vi "PathPlanner_Cmd_AutoRamseteExecute.vi"(5 "PathPlanner_Cmd_FollowRamConfig":T18={"ControlPastEnd_Sec"=3.0, "Trigger Events"=TRUE, "RAMSETE_EXE_TUNING SI"={"B"=2.0, "Zeta"=0.7, "X Tolerance M"=2.0, "Y Tolerance M"=0.7, "Heading Tolerance RAD"=0.7, "Track Width M"=2.0, "Max Speed M/S"=2.0}} {"RAMSETE_EXE_TUNING SI"."Max Speed M/S" format="%13.4f"; "RAMSETE_EXE_TUNING SI"."Track Width M" format="%13.4f"; "RAMSETE_EXE_TUNING SI"."Heading Tolerance RAD" format="%13.4f"; "RAMSETE_EXE_TUNING SI"."Y Tolerance M" format="%13.4f"; "RAMSETE_EXE_TUNING SI"."X Tolerance M" format="%13.4f"; "RAMSETE_EXE_TUNING SI"."Zeta" format="%13.4f"; "RAMSETE_EXE_TUNING SI"."B" format="%13.4f"}, 6 "PassthroughTime_SEC":dbl=-1.0, 7 "PathPlanner_Cmd_AutoConfig":T3 {"Paths"."IdealStartingState"."Rotation"."SIN" format="%13.4f"; "Paths"."IdealStartingState"."Rotation"."COS" format="%13.4f"; "Paths"."IdealStartingState"."Rotation"."VALUE" format="%13.4f"; "Paths"."PointTowardsZones"."TargetPosition"."Y" format="%14.3f"; "Paths"."PointTowardsZones"."TargetPosition"."X" format="%14.3f"; "Paths"."PointTowardsZones"."RotationOffset"."SIN" format="%13.4f"; "Paths"."PointTowardsZones"."RotationOffset"."COS" format="%13.4f"; "Paths"."PointTowardsZones"."RotationOffset"."VALUE" format="%13.4f"; "Paths"."Waypoints"."nextControl"."Y" format="%14.3f"; "Paths"."Waypoints"."nextControl"."X" format="%14.3f"; "Paths"."Waypoints"."anchor"."Y" format="%14.3f"; "Paths"."Waypoints"."anchor"."X" format="%14.3f"; "Paths"."Waypoints"."prevControl"."Y" format="%14.3f"; "Paths"."Waypoints"."prevControl"."X" format="%14.3f"; "Paths"."AllPoints"."RotationTarget"."rotation"."SIN" format="%13.4f"; "Paths"."AllPoints"."RotationTarget"."rotation"."COS" format="%13.4f"; "Paths"."AllPoints"."RotationTarget"."rotation"."VALUE" format="%13.4f"; "Paths"."AllPoints"."Position"."Y" format="%14.3f"; "Paths"."AllPoints"."Position"."X" format="%14.3f"; "Paths"."GoalEndState"."Rotation"."SIN" format="%13.4f"; "Paths"."GoalEndState"."Rotation"."COS" format="%13.4f"; "Paths"."GoalEndState"."Rotation"."VALUE" format="%13.4f"; "Paths"."RotationTargets"."rotation"."SIN" format="%13.4f"; "Paths"."RotationTargets"."rotation"."COS" format="%13.4f"; "Paths"."RotationTargets"."rotation"."VALUE" format="%13.4f"}, 8 "Enabled":bool=TRUE, 9 "Reset":bool, 10 "CurrentChassisSpeeds":T2 {"vOmega" format="%10.3f"; "vY" format="%10.3f"; "vX" format="%10.3f"}, 11 "Current Pose SI":T20={"TRANSLATION"={"X"=0.0, "Y"=0.0}, "ROTATION"={"VALUE"=0.0, "COS"=1.0, "SIN"=0.0}} {"ROTATION"."SIN" format="%13.4f"; "ROTATION"."COS" format="%13.4f"; "ROTATION"."VALUE" format="%13.4f"; "TRANSLATION"."Y" format="%14.3f"; "TRANSLATION"."X" format="%14.3f"}) -> (0 "Position Error M":dbl, 1 "Complete":bool, 2 "At Reference":bool, 3 "Left Right Speed Dmds":T1)   [LabVIEW 2019, in "PathPlanner24.lvlib"]
doc: "DOCUMENTATION IS NOT COMPLETE.\n \nCalculates the next output of the path following controller for holonomic drive robots. This wraps a Holonomic Drive Control function with the particulars needed to follow a PathPlanner trajectory.\n\nInputs:\n - PathPlanner_Holonomic_Ctrl_Pack_Tuning - cluster - The tuning paraameters for the holonomic drive controller. These are static. They should not be changed after the first call to this function.\n - CurrentPoseSi - pose2d - The current pose calculated by odometry or pose estimation. The pose can be absolute or relative depending on what type of trajectory is being followed.\n - PathPlannerState - cluster - The path palnner trajectory state containing the desired position and velocities of the robot.\n - Reset - boolean - When TRUE the holonomic drive controller is reset. This should be set to TRUE for the first execution of a trajectory.\n - Enabled - boolean - When TRUE, closed loop control is enabled. (Optional. Default: TRUE)\n - Period - double - The loop period in seconds for this controller. (Optional. Default: 0.020)\n\nOutputs:\n - CalcChassisSpeed - cluster - The desired chassis speed in SI units.\n - AtReference - boolean - TRUE if the robots position is within the defined tolerance.\n - PositionError - pose2d - Position error in SI units. How far the robot is away from the desired trajectory position.\n - out_Holonomic_Drive_Ctrl - THe current holonomic drive controller data cluster. This is mainly for diagnostic purposes."
uses:
  PathPlanner24.lvlib
  <vilib>/Rock Robotics/WPI/ThirdParty/JAS_Junk/TrajLib/TypeDef/TRANSLATION2D.ctl
  <vilib>/Rock Robotics/WPI/ThirdParty/JAS_Junk/TrajLib/Trajectory_Library.lvlib
  <vilib>/Rock Robotics/WPI/ThirdParty/JAS_Junk/TrajLib/TypeDef/ROTATION2D.ctl
  <vilib>/Rock Robotics/WPI/ThirdParty/JAS_Junk/TrajLib/TypeDef/POSE2D.ctl
  <vilib>/Rock Robotics/WPI/ThirdParty/JAS_Junk/TrajLib/TypeDef/CHASSIS_SPEEDS.ctl
  TypeDef/PathPlannerRotationTarget.ctl
  TypeDef/PathPlannerPathConstraints.ctl
  TypeDef/PathPlannerConstraintsZone.ctl
  TypeDef/PathPlannerCommandUtil.ctl
  TypeDef/PathPlannerEventMarker.ctl
  TypeDef/PathPlannerGoalEndState.ctl
  TypeDef/PathPlannerPathPoint.ctl
  TypeDef/PathPlannerPath.ctl
  TypeDef/PathPlannerWaypoint.ctl
  TypeDef/PathPlannerPointTowardsZone.ctl
  TypeDef/PathPlannerIdealStartingState.ctl
  TypeDef/PathPlannerCmdPathPlannerAutoConfig.ctl
  <vilib>/Rock Robotics/WPI/ThirdParty/JAS_Junk/TrajLib/TypeDef/RAMSETE_EXE_TUNING.ctl
  TypeDef/PathPlannerCmdFollowRamConfig.ctl
  ENum/PathPlanner_CommandUtil_Type_ENUM.ctl
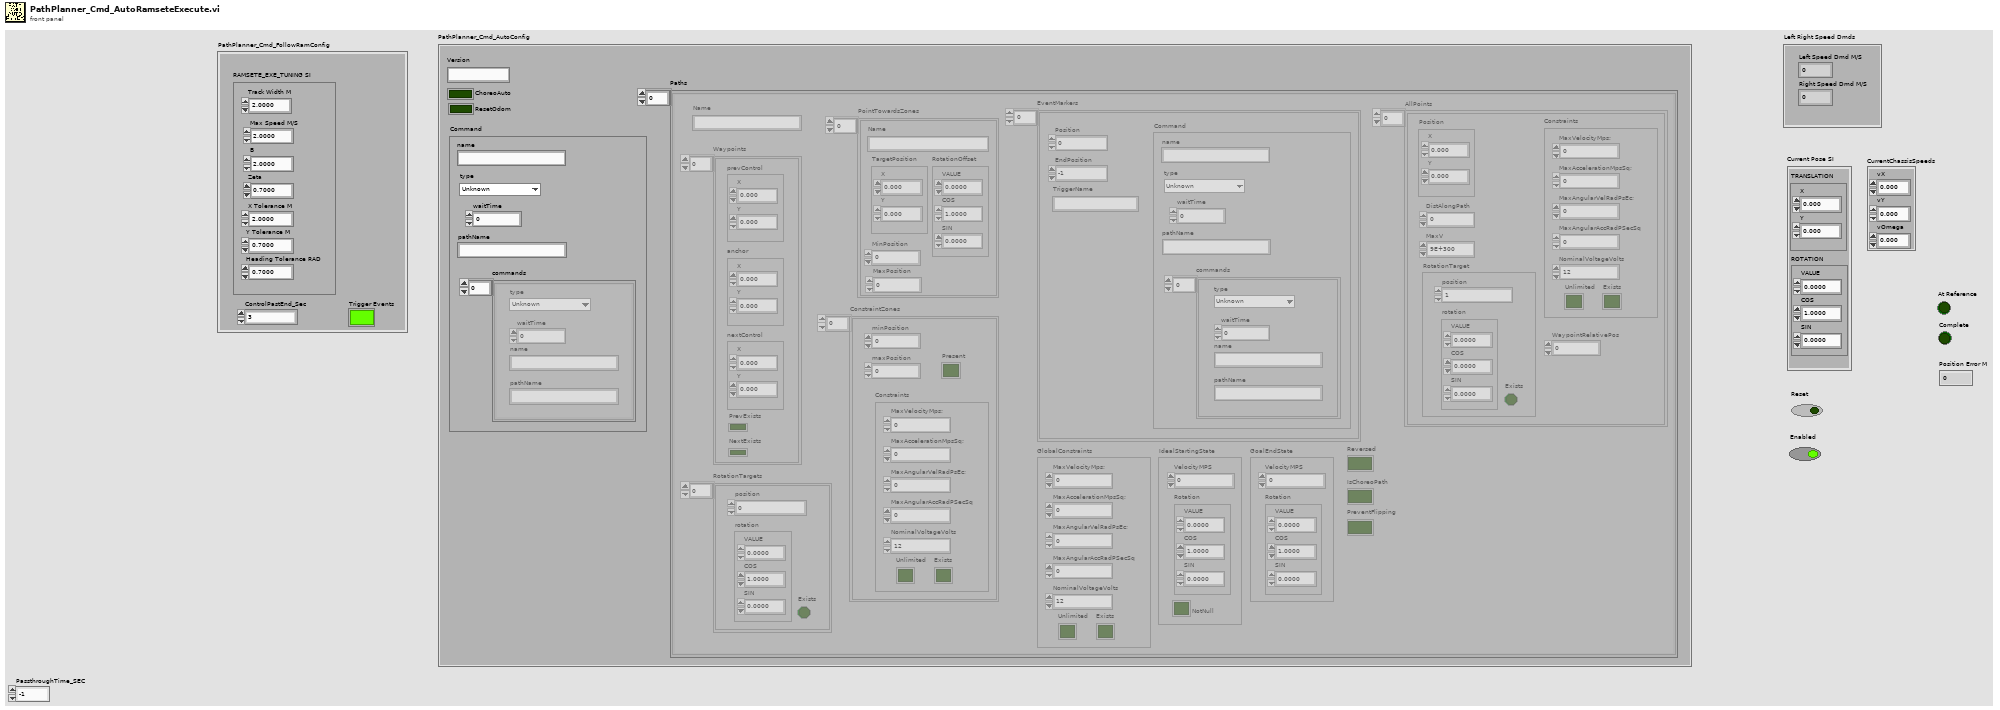
[diagram p1: front panel]
types:
  T1 = cluster{"Left Speed Dmd M/S":dbl, "Right Speed Dmd M/S":dbl}
  T2 = typedef "Trajectory_Library.lvlib/CHASSIS_SPEEDS.ctl" = cluster{"vX":dbl, "vY":dbl, "vOmega":dbl}
  T3 = typedef "PathPlanner24.lvlib/PathPlannerCmdPathPlannerAutoConfig.ctl" = cluster{"Command":T4, "ChoreoAuto":bool, "Version":string, "ResetOdom":bool, "Paths":T6[]}
  T4 = typedef "PathPlanner24.lvlib/PathPlannerCommandUtil.ctl" = cluster{"waitTime":dbl, "name":string, "pathName":string, "commands":cluster{"type":T5, "waitTime":dbl, "name":string, "pathName":string}[], "type":T5}
  T5 = typedef "PathPlanner24.lvlib/PathPlanner_CommandUtil_Type_ENUM.ctl" = enum16{"Unknown", "Wait", "Named", "Path", "Sequential", "Parallel", "Race", "Deadline", "PointTowardsZoneEnter", "PointTowardsZoneExit", "TriggerEventStart", "TriggerEventStop", "TriggerEventOneshot"}
  T6 = typedef "PathPlanner24.lvlib/PathPlannerPath.ctl" = cluster{"Reversed":bool, "RotationTargets":T7[], "ConstraintZones":T9[], "EventMarkers":T11[], "GlobalConstraints":T10, "GoalEndState":T12, "AllPoints":T13[], "Name":string, "Waypoints":T15[], "PointTowardsZones":T16[], "IdealStartingState":T17, "IsChoreoPath":bool, "PreventFlipping":bool}
  T7 = typedef "PathPlanner24.lvlib/PathPlannerRotationTarget.ctl" = cluster{"position":dbl, "rotation":T8, "Exists":bool}
  T8 = typedef "Trajectory_Library.lvlib/ROTATION2D.ctl" = cluster{"VALUE":dbl, "COS":dbl, "SIN":dbl}
  T9 = typedef "PathPlanner24.lvlib/PathPlannerConstraintsZone.ctl" = cluster{"minPosition":dbl, "maxPosition":dbl, "Constraints":T10, "Present":bool}
  T10 = typedef "PathPlanner24.lvlib/PathPlannerPathConstraints.ctl" = cluster{"MaxVelocityMps;":dbl, "MaxAccelerationMpsSq;":dbl, "MaxAngularVelRadPsEc;":dbl, "MaxAngularAccRadPSecSq":dbl, "Exists":bool, "Unlimited":bool, "NominalVoltageVolts":dbl}
  T11 = typedef "PathPlanner24.lvlib/PathPlannerEventMarker.ctl" = cluster{"Position":dbl, "Command":T4, "TriggerName":string, "EndPosition":dbl}
  T12 = typedef "PathPlanner24.lvlib/PathPlannerGoalEndState.ctl" = cluster{"VelocityMPS":dbl, "Rotation":T8}
  T13 = typedef "PathPlanner24.lvlib/PathPlannerPathPoint.ctl" = cluster{"Position":T14, "DistAlongPath":dbl, "MaxV":dbl, "Constraints":T10, "RotationTarget":T7, "WaypointRelativePos":dbl}
  T14 = typedef "Trajectory_Library.lvlib/TRANSLATION2D.ctl" = cluster{"X":dbl, "Y":dbl}
  T15 = typedef "PathPlanner24.lvlib/PathPlannerWaypoint.ctl" = cluster{"prevControl":T14, "anchor":T14, "nextControl":T14, "PrevExists":bool, "NextExists":bool}
  T16 = typedef "PathPlanner24.lvlib/PathPlannerPointTowardsZone.ctl" = cluster{"RotationOffset":T8, "Name":string, "TargetPosition":T14, "MinPosition":dbl, "MaxPosition":dbl}
  T17 = typedef "PathPlanner24.lvlib/PathPlannerIdealStartingState.ctl" = cluster{"VelocityMPS":dbl, "Rotation":T8, "NotNull":bool}
  T18 = typedef "PathPlanner24.lvlib/PathPlannerCmdFollowRamConfig.ctl" = cluster{"ControlPastEnd_Sec":dbl, "Trigger Events":bool, "RAMSETE_EXE_TUNING SI":T19}
  T19 = typedef "Trajectory_Library.lvlib/RAMSETE_EXE_TUNING.ctl" = cluster{"B":dbl, "Zeta":dbl, "X Tolerance M":dbl, "Y Tolerance M":dbl, "Heading Tolerance RAD":dbl, "Track Width M":dbl, "Max Speed M/S":dbl}
  T20 = typedef "Trajectory_Library.lvlib/POSE2D.ctl" = cluster{"TRANSLATION":T14, "ROTATION":T8}
  T21 = cluster{"type":T5, "waitTime":dbl, "name":string, "pathName":string}[]
  T22 = cluster{"type":T5, "waitTime":dbl, "name":string, "pathName":string}
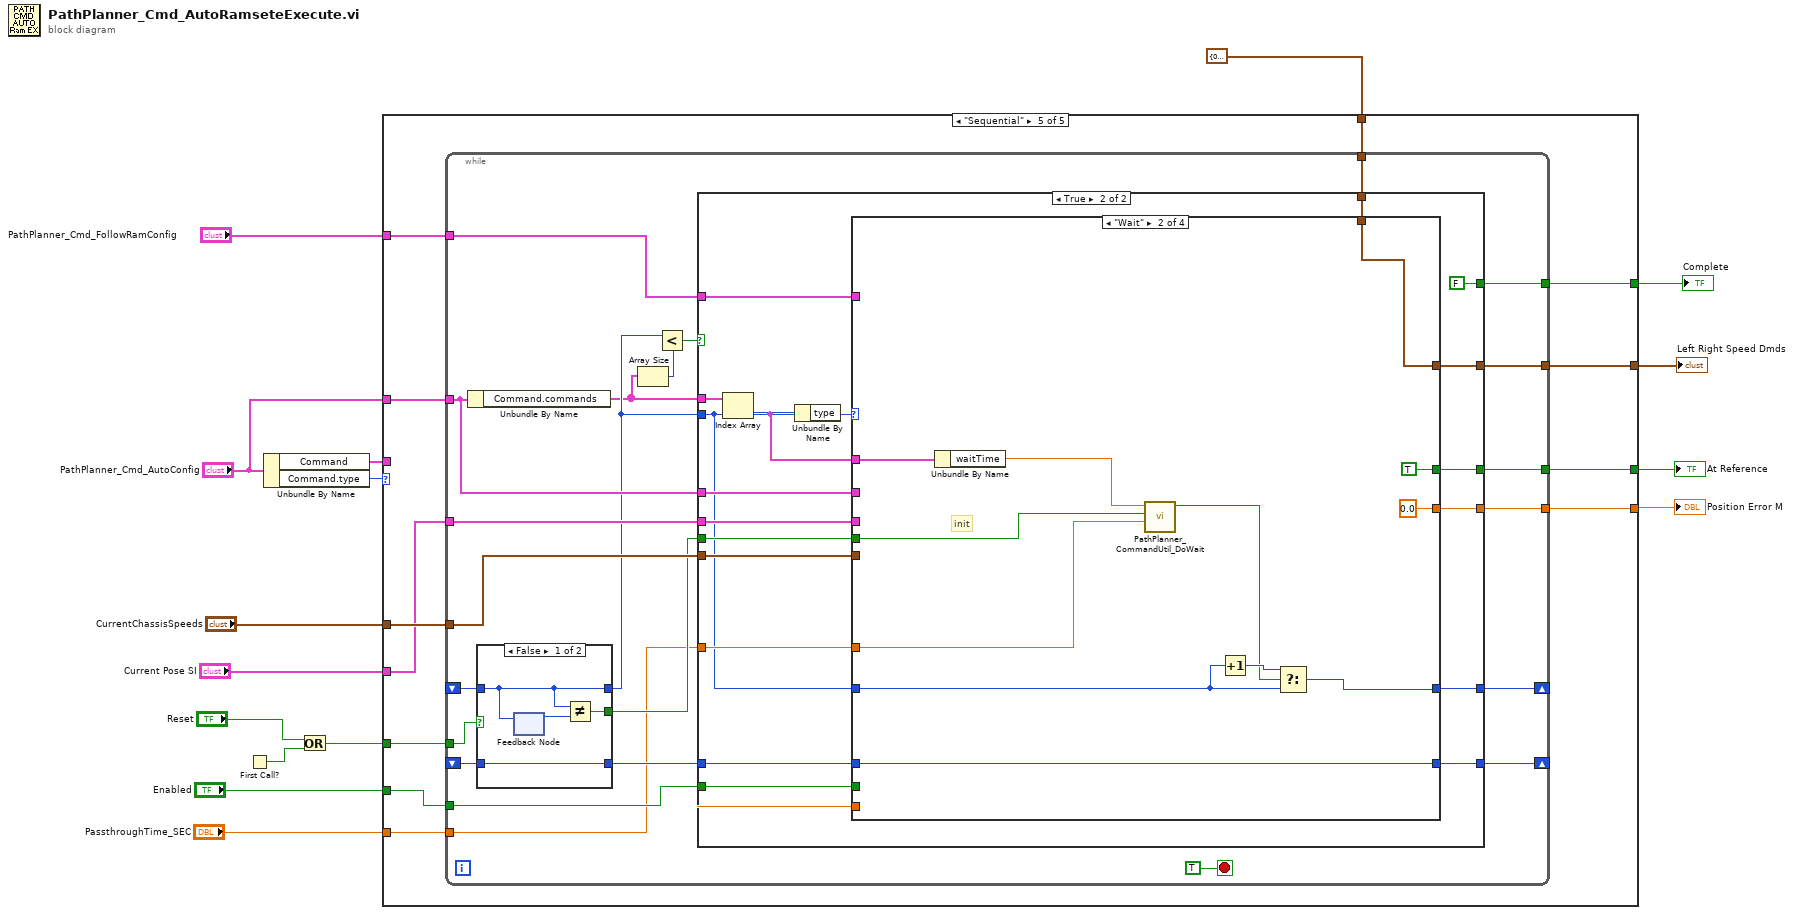
[diagram p0: block diagram]
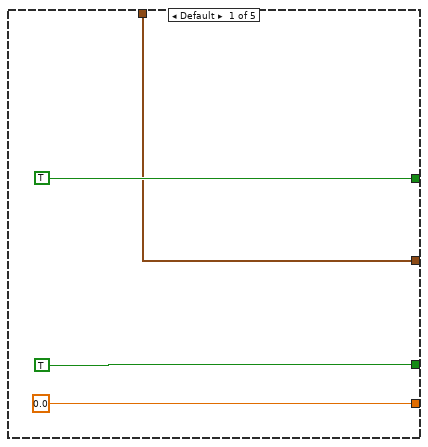
[diagram p2: hidden frame]
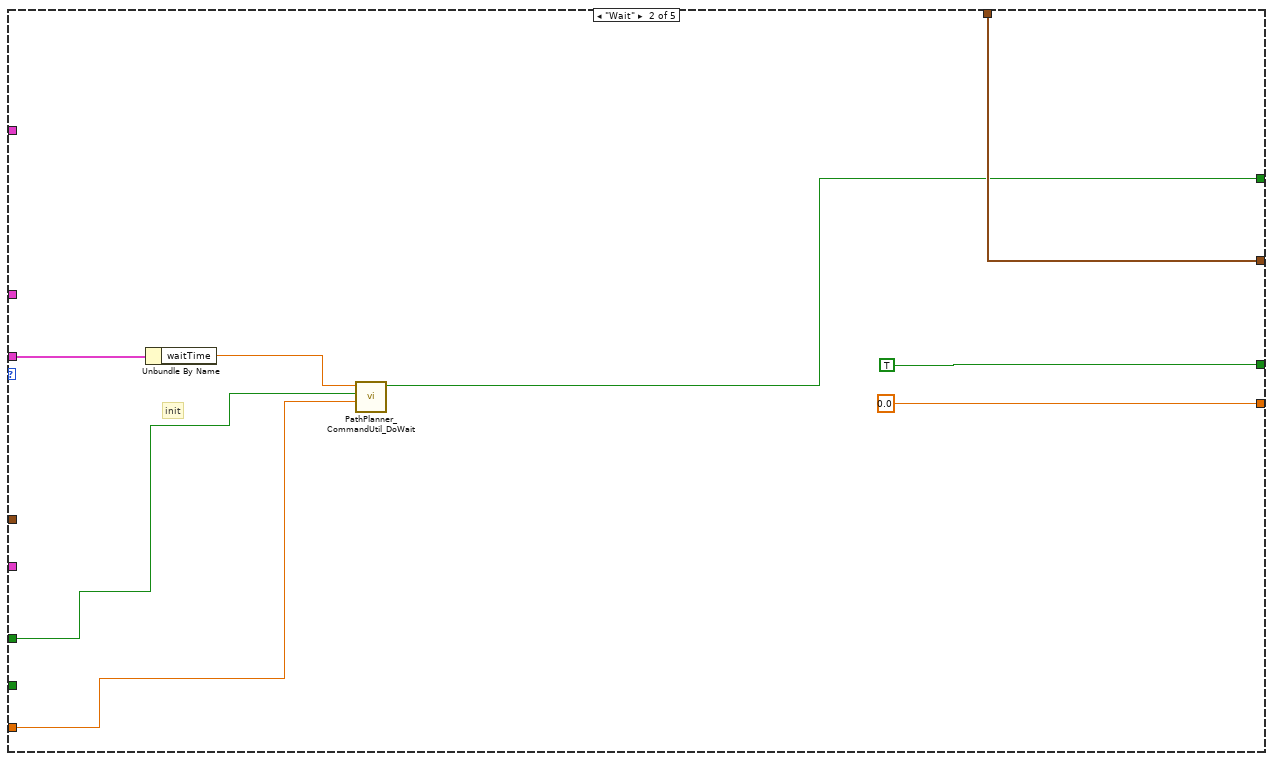
[diagram p3: hidden frame]
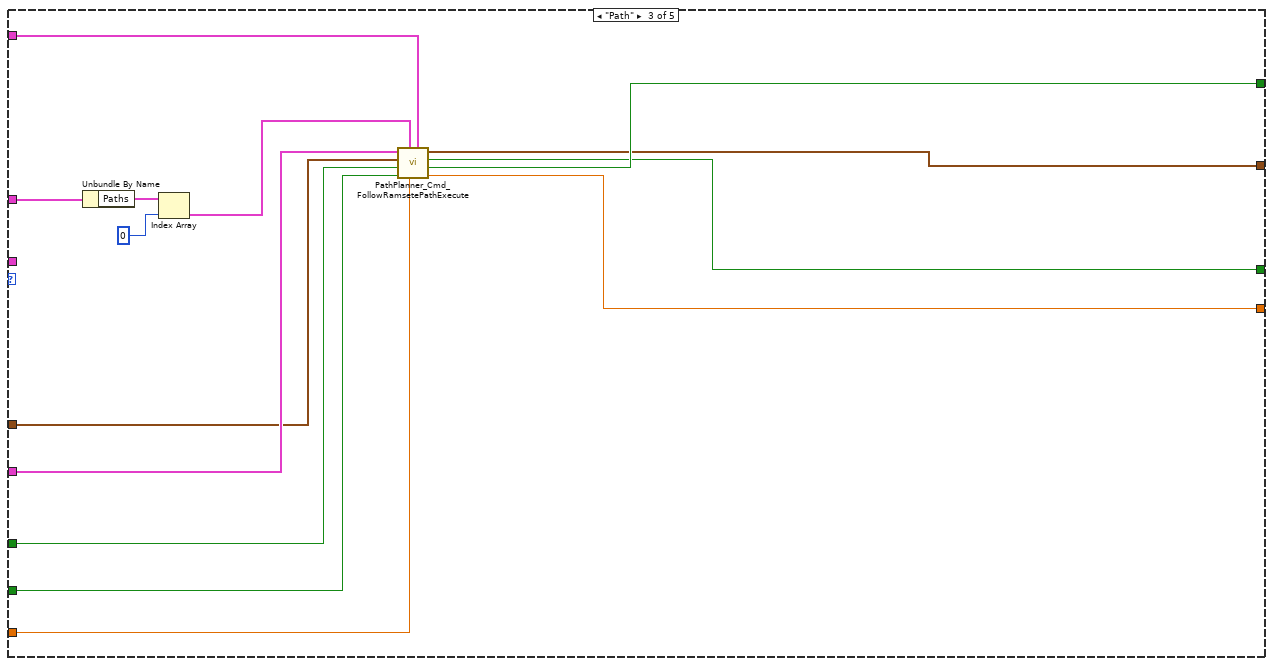
[diagram p4: hidden frame]
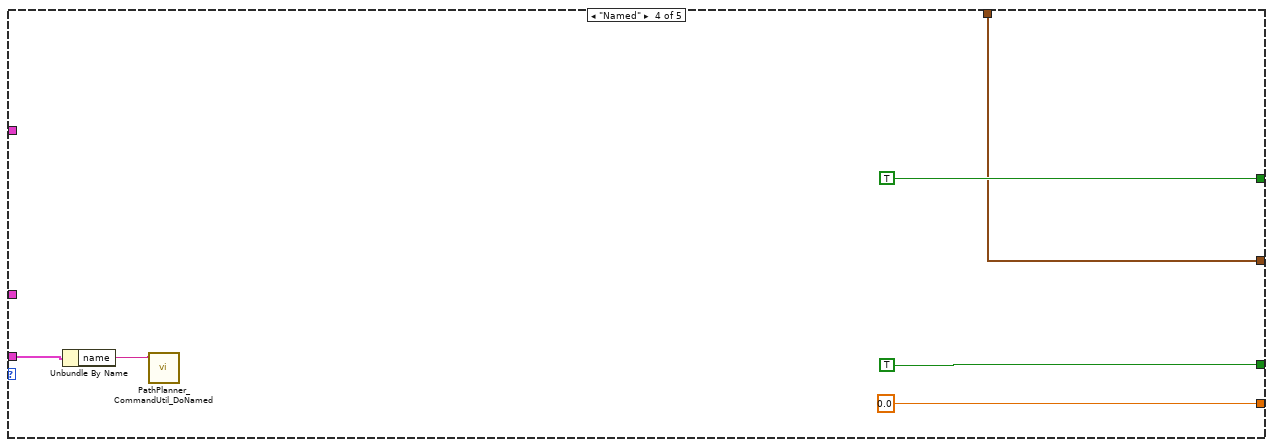
[diagram p5: hidden frame]
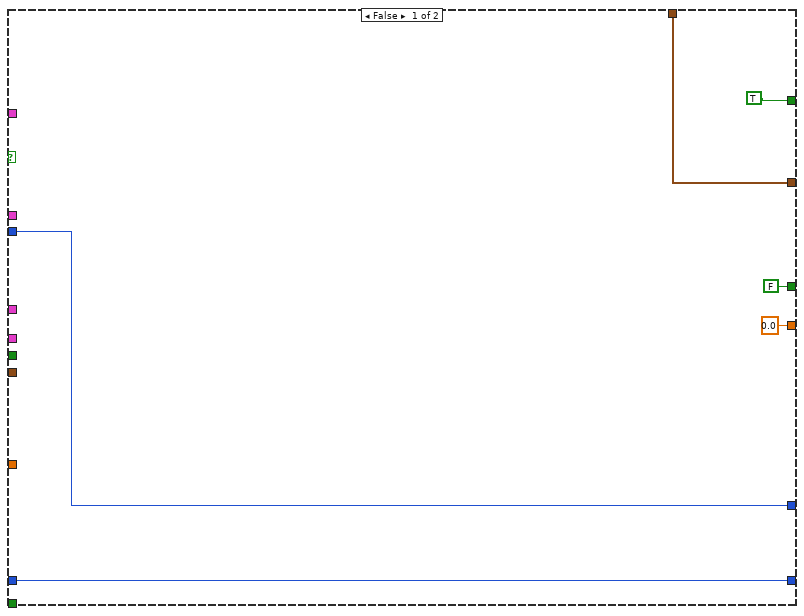
[diagram p6: hidden frame]
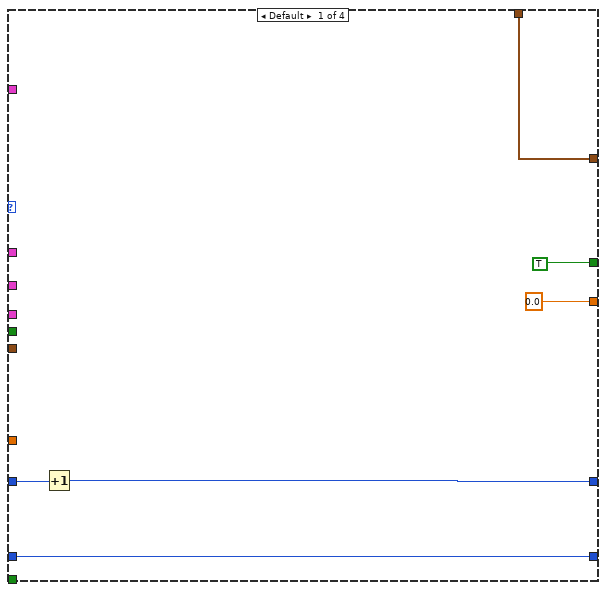
[diagram p7: hidden frame]
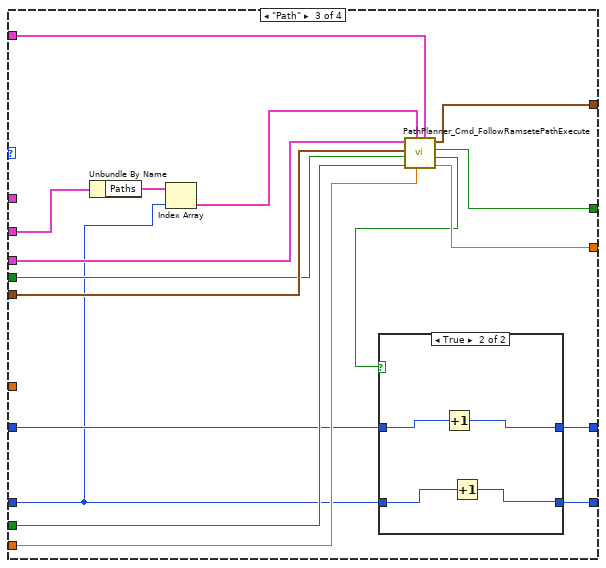
[diagram p8: hidden frame]
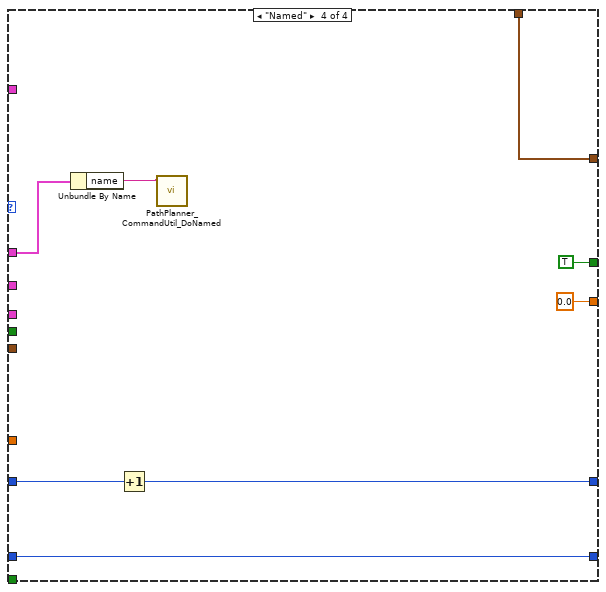
[diagram p10: hidden frame]
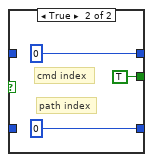
[diagram p11: hidden frame]
diagram:
  n1 = First Call?() -> (First Call?: T/F=w15:bool)
  n2 = Unbundle By Name("PathPlanner_Cmd_AutoConfig") -> ("Command"=w13:T4, "Command.type"=w14:T5)
  n3 = Or(x="Reset", y=w15) -> (x .or. y?=w8:bool)
  n4 = case shown="\"Sequential\"" w14 {
    tunnel: w13 -> [_ w24 _ w43 _]
    tunnel: "PathPlanner_Cmd_AutoConfig" -> [_ _ w42 _ w59]
    tunnel: "PathPlanner_Cmd_FollowRamConfig" -> [_ _ w38 _ w53]
    tunnel: "Current Pose SI" -> [_ _ w37 _ w52]
    tunnel: "CurrentChassisSpeeds" -> [_ _ w36 _ w58]
    tunnel: w8 -> [_ w23 w35 _ w60]
    tunnel: "Enabled" -> [_ _ w34 _ w51]
    tunnel: "PassthroughTime_SEC" -> [_ w22 w33 _ w55]
    tunnel: [0.0 ("Position Error M") 0.0 ("Position Error M") w32 0.0 ("Position Error M") w56] -> w5
    tunnel: [TRUE ("Complete") w21 w31 TRUE ("Complete") w50] -> w4
    tunnel: [TRUE ("At Reference") TRUE ("At Reference") w30 TRUE ("At Reference") w57] -> w3
    tunnel: T1 {"Left Speed Dmd M/S"=0.0, "Right Speed Dmd M/S"=0.0} ("Left Right Speed Dmds") -> [w17 w26 _ w45 w54]
    tunnel: [w17 w26 w29 w45 w49] -> w2
    frame Default {
    }
    frame "Wait" {
      # "init"
      n5 = Unbundle By Name(w24) -> ("waitTime"=w25:dbl)
      n6 = call "PathPlanner_CommandUtil_DoWait.vi"("PassthroughTime_SEC"=w22, "Init"=w23, "WaitTimeSec"=w25) -> ("Done"=w21:bool)  [unwired: 8 in]
    }
    frame "Path" {
      n7 = Unbundle By Name(w42) -> ("Paths"=w41:T6[])
      n8 = Index Array(array=w41, index=0) -> (element=w39:T6)
      n9 = call "PathPlanner_Cmd_FollowRamsetePathExecute.vi"("PathPlanner_Cmd_FollowRamConfig"=w38, "PassthroughTime_SEC"=w33, "PathPlannerPath"=w39, "Enabled"=w34, "Reset"=w35, "CurrentChassisSpeeds"=w36, "Current Pose SI"=w37) -> ("Position Error M"=w32:dbl, "Complete"=w31:bool, "At Reference"=w30:bool, "Left Right Speed Dmds"=w29:T1)  [unwired: 1 out]
    }
    frame "Named" {
      n10 = Unbundle By Name(w43) -> ("name"=w44:string)
      n11 = call "PathPlanner_CommandUtil_DoNamed.vi"("Event Action Name"=w44) -> ()  [unwired: 11 in]
    }
    frame "Sequential" {
      n12 = while {
        tunnel: w60 -> [w79]
        tunnel: w59 -> [w74]
        tunnel: w58 -> [w82]
        tunnel: [w81] -> w57
        tunnel: [w80] -> w56
        tunnel: w55 -> [w69]
        shift-right: [w68] -> _
        shift-left: _ -> [w78]
        shift-right: [w67] -> _
        shift-left: _ -> [w77]
        tunnel: w54 -> [w75]
        tunnel: w53 -> [w72]
        tunnel: w52 -> [w71]
        tunnel: w51 -> [w70]
        tunnel: [w62] -> w50
        tunnel: [w61] -> w49
        stop <- TRUE stop-if-true
        n13 = Unbundle By Name(w74) -> ("Command.commands"=w64:T21)
        n14 = case shown="False" w79 {
          tunnel: [w158 0] -> w66
          tunnel: [w160 0] -> w73
          tunnel: w78 -> [w158 _]
          tunnel: w77 -> [w160 _]
          tunnel: [w161 TRUE] -> w76
          frame False {
            n15 = feedback-in #1(w158) -> ()
            n16 = feedback #1() -> (w159:i32)  [unwired: 1 in]
            n17 = Not Equal?(x=w158, y=w159) -> (x != y?=w161:bool)
          }
          frame True {
            # "path index"
            # "cmd index"
          }
        }
        n18 = Array Size(array=w64) -> (size(s)=w65:i32)
        n19 = Less?(x=w66, y=w65) -> (x < y?=w63:bool)
        n20 = case shown="True" w63 {
          tunnel: w82 -> [_ w108]
          tunnel: [FALSE ("At Reference") w107] -> w81
          tunnel: [0.0 ("Position Error M") w106] -> w80
          tunnel: w64 -> [_ w105]
          tunnel: w76 -> [_ w103]
          tunnel: w75 -> [w84 w101]
          tunnel: w74 -> [_ w100]
          tunnel: w73 -> [w85 w99]
          tunnel: w72 -> [_ w98]
          tunnel: w71 -> [_ w97]
          tunnel: w70 -> [_ w96]
          tunnel: w69 -> [_ w95]
          tunnel: w66 -> [w86 w91]
          tunnel: [w86 w94] -> w68
          tunnel: [w85 w93] -> w67
          tunnel: [TRUE FALSE] -> w62
          tunnel: [w84 w90] -> w61
          frame False {
          }
          frame True {
            n21 = Index Array(array=w105, index=w91) -> (element=w102:T22)
            n22 = Unbundle By Name(w102) -> ("type"=w104:T5)
            n23 = case shown="\"Wait\"" w104 {
              tunnel: w108 -> [_ _ w138 _]
              tunnel: [TRUE TRUE ("At Reference") w134 TRUE ("At Reference")] -> w107
              tunnel: [0.0 0.0 ("Position Error M") w133 0.0 ("Position Error M")] -> w106
              tunnel: w95 -> [_ w117 _ _]
              tunnel: w103 -> [_ w118 w137 _]
              tunnel: w102 -> [_ w119 _ w157]
              tunnel: w101 -> [w109 w123 _ w151]
              tunnel: w100 -> [_ _ w141 _]
              tunnel: w99 -> [w110 w126 w130 w152]
              tunnel: w98 -> [_ _ w140 _]
              tunnel: w97 -> [_ _ w139 _]
              tunnel: w96 -> [_ _ w136 _]
              tunnel: w95 -> [_ _ w135 _]
              tunnel: w91 -> [w112 w116 w131 w154]
              tunnel: [w111 w115 w128 w153] -> w94
              tunnel: [w110 w126 w129 w152] -> w93
              tunnel: [w109 w123 w127 w151] -> w90
              frame Default {
                n24 = Increment(x=w112) -> (x+1=w111:i32)
              }
              frame "Wait" {
                # "init"
                n25 = Unbundle By Name(w119) -> ("waitTime"=w122:dbl)
                n26 = call "PathPlanner_CommandUtil_DoWait.vi"("PassthroughTime_SEC"=w117, "Init"=w118, "WaitTimeSec"=w122) -> ("Done"=w120:bool)  [unwired: 8 in]
                n27 = Increment(x=w116) -> (x+1=w121:i32)
                n28 = Select(t=w121, s=w120, f=w116) -> (s? t:f=w115:i32)
              }
              frame "Path" {
                n29 = Unbundle By Name(w141) -> ("Paths"=w143:T6[])
                n30 = Index Array(array=w143, index=w130) -> (element=w142:T6)
                n31 = call "PathPlanner_Cmd_FollowRamsetePathExecute.vi"("PathPlanner_Cmd_FollowRamConfig"=w140, "PassthroughTime_SEC"=w135, "PathPlannerPath"=w142, "Enabled"=w136, "Reset"=w137, "CurrentChassisSpeeds"=w138, "Current Pose SI"=w139) -> ("Position Error M"=w133:dbl, "Complete"=w132:bool, "At Reference"=w134:bool, "Left Right Speed Dmds"=w127:T1)  [unwired: 1 out]
                n32 = case shown="True" w132 {
                  tunnel: w131 -> [w144 w149]
                  tunnel: w130 -> [w145 w147]
                  tunnel: [w145 w146] -> w129
                  tunnel: [w144 w148] -> w128
                  frame False {
                  }
                  frame True {
                    n33 = Increment(x=w149) -> (x+1=w148:i32)
                    n34 = Increment(x=w147) -> (x+1=w146:i32)
                  }
                }
              }
              frame "Named" {
                n35 = Unbundle By Name(w157) -> ("name"=w150:string)
                n36 = Increment(x=w154) -> (x+1=w153:i32)
                n37 = call "PathPlanner_CommandUtil_DoNamed.vi"("Event Action Name"=w150) -> ()  [unwired: 11 in]
              }
            }
          }
        }
      }
    }
  }
  "At Reference" <- w3
  "Position Error M" <- w5
  "Complete" <- w4
  "Left Right Speed Dmds" <- w2
